vi "Get_Groups_And_Names.vi"(8 "error in (no error)":errorcluster, 11 "Constraints":T1 {"Estimate Quality" scale=0.0..5.0}) -> (0 "error out":errorcluster, 1 "Description":string[](array[string]), 2 "Groups":string[](array[string]), 3 "Names":string[](array[string]), 4 "Description Returned?":bool, 5 "Run start integer timestamp":i64[](array[numeric]), 6 "Run Time (hrs)":string[](array[string]), 7 "Run stop integer timestamp":i64[](array[numeric]))   [LabVIEW 2013]
uses:
  Constraints.ctl
  <vilib>/addons/database/Auxilliary.llb/DB Tools Cursor Type.ctl
  <vilib>/addons/database/Connection.llb/Conn Execute.vi
  <vilib>/addons/database/Recordset.llb/Rec Fetch Recordset Data (R).vi
  <userlib>/_OpenG.lib/array/array.llb/Empty 2D Array (Variant)__ogtk.vi
  <vilib>/addons/database/Recordset.llb/Rec Destroy - Connection.vi
  <userlib>/_OpenG.lib/array/array.llb/Remove Duplicates from 1D Array (String)__ogtk.vi
  <vilib>/addons/database/_DB Variant To Data/Database Variant To Data.xnode
  <vilib>/addons/database/NI_Database_API.lvlib
panel:
  out "SQL Lower Settings Query":string
  out "SQL Upper Settings Query":string
  out "Names SQL Query":string
  out "Groups SQL Query":string
  out "resulting string":string
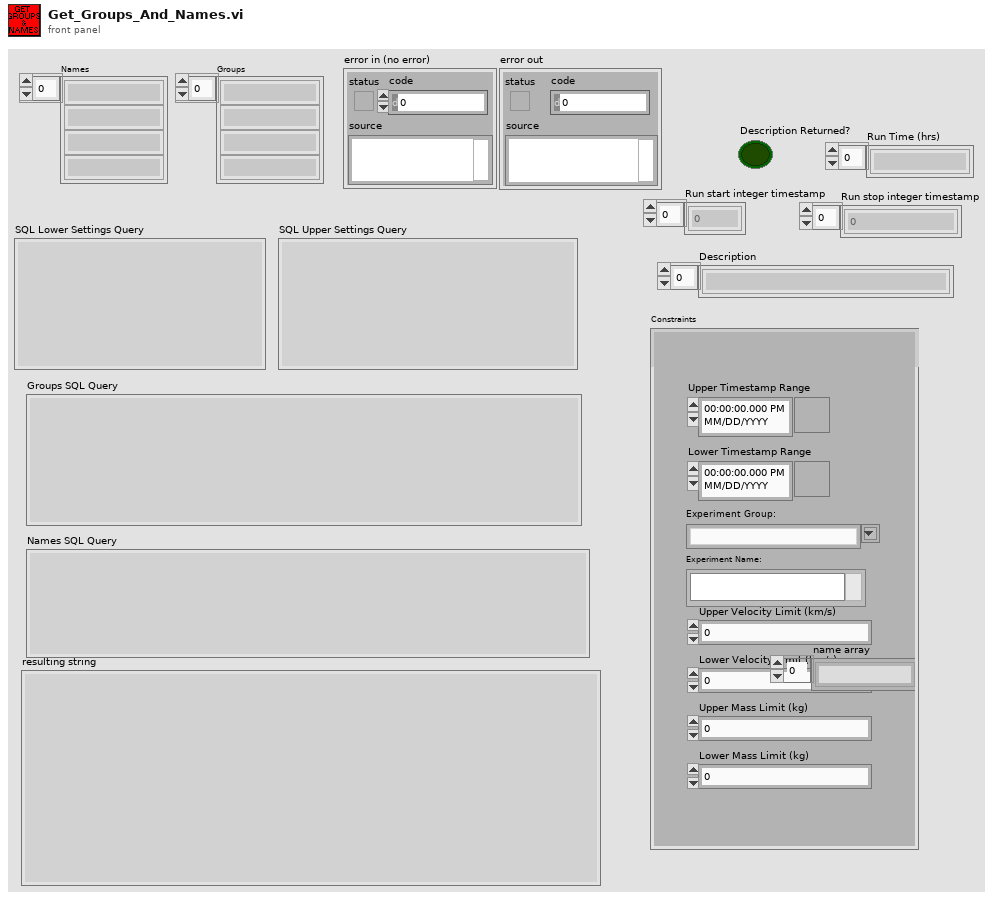
[diagram p1: front panel]
types:
  T1 = typedef "Constraints.ctl" = cluster{"Upper Timestamp Range":timestamp, "Lower Timestamp Range":timestamp, "Experiment Group:":string, "Experiment Name:":i32[], "Upper Velocity Limit (km/s)":dbl, "Lower Velocity Limit (km/s)":dbl, "Upper Mass Limit (kg)":dbl, "Lower Mass Limit (kg)":dbl, "name array":string[], "Estimate Quality":cluster{dbl, dbl}}
  T2 = typedef "NI_Database_API.lvlib/DB Tools Cursor Type.ctl" = enum16{"forward-only", "keyset", "dynamic", "static"}
  T3 = typedef "NI_Database_API.lvlib/Conn ObjectReference.ctl" = refnum<k1>
  T4 = typedef "NI_Database_API.lvlib/Rec ObjectReference.ctl" = refnum<k1>
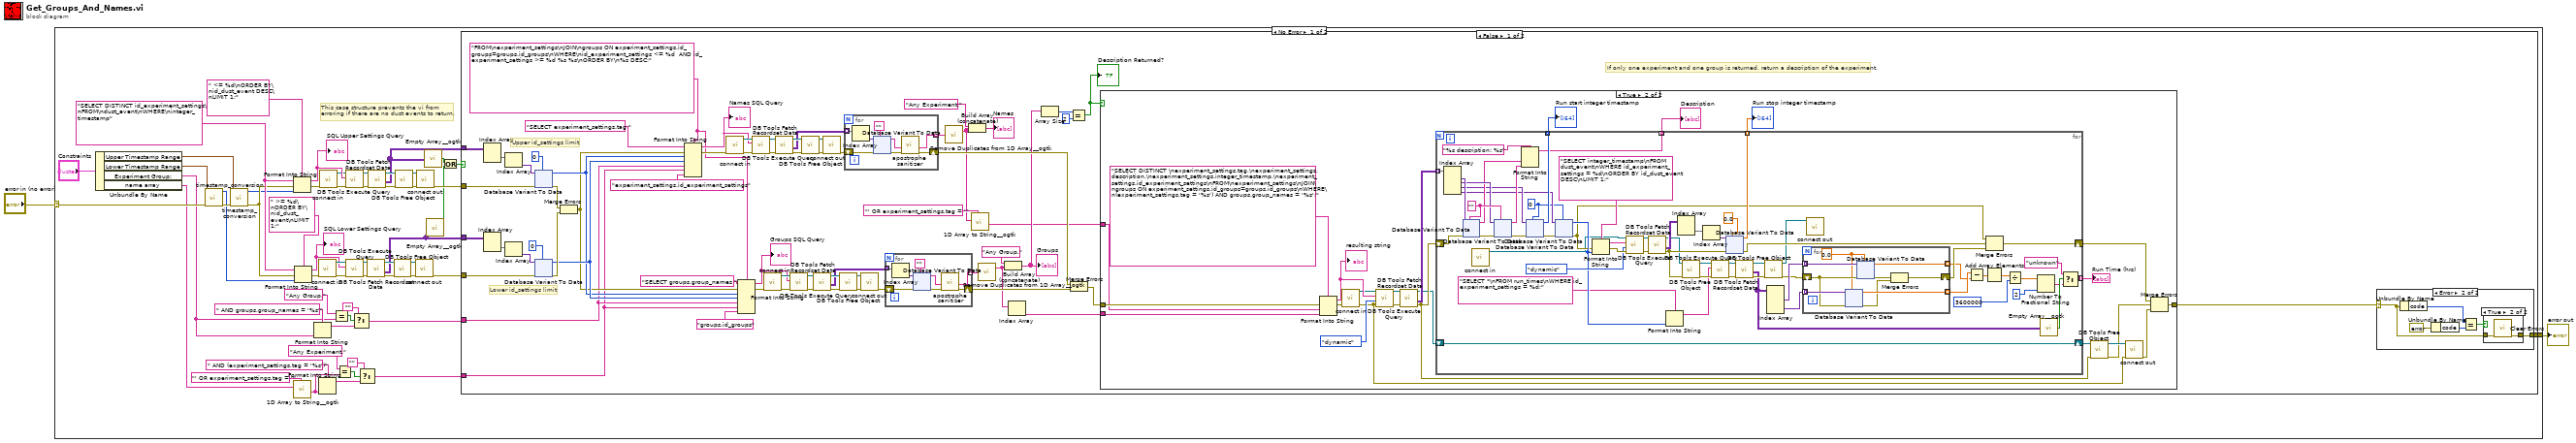
[diagram p0: block diagram]
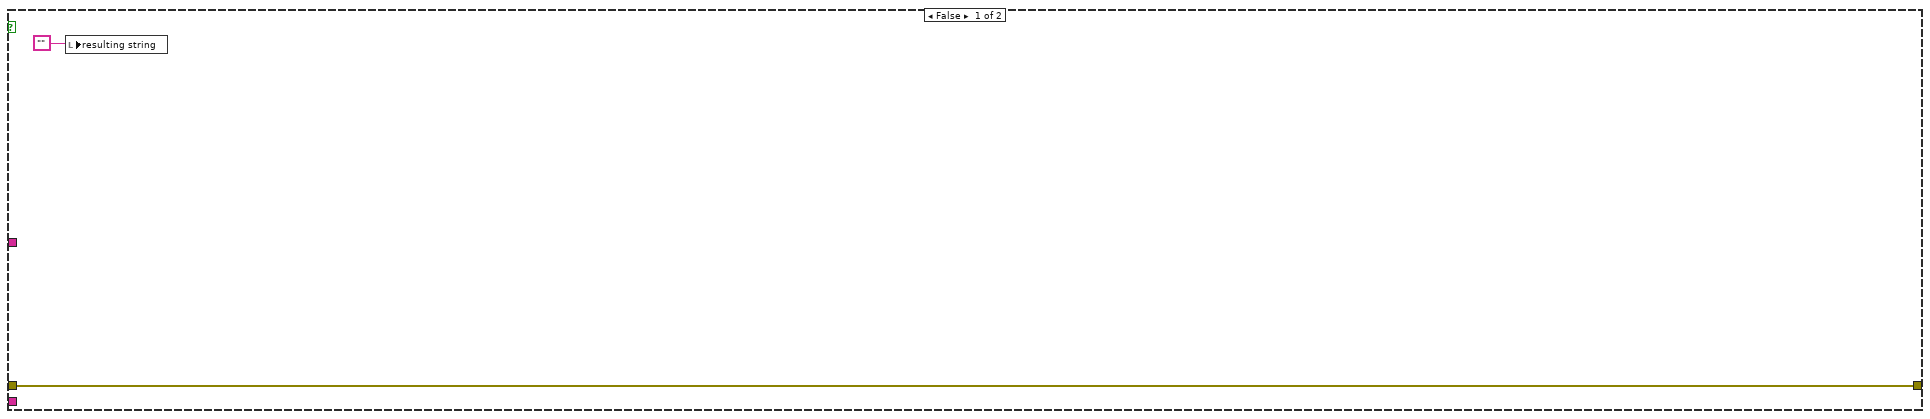
[diagram p4: hidden frame]
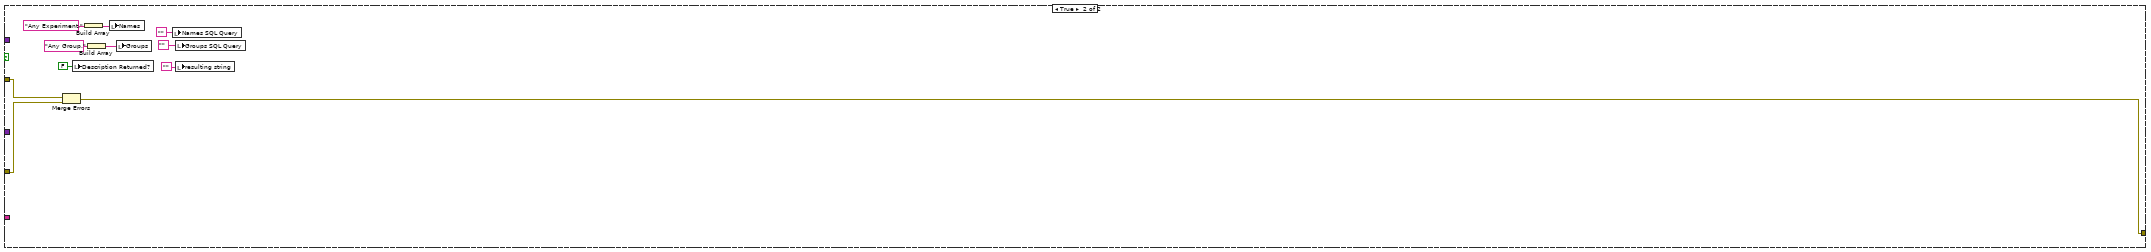
[diagram p5: hidden frame]
diagram:
  n1 = case shown="No Error" "error in (no error)" {
    selector: "error in (no error)" -> [w53 w607]
    tunnel: [w57 w607] -> w2
    frame No Error {
      w49 = "SELECT DISTINCT id_experiment_settings\nFROM\ndust_event\nWHERE\ninteger_timestamp" ("format string")
      # "This case structure prevents the vi from\nerroring if there are no dust events to return."
      n2 = Unbundle By Name("Constraints") -> ("Upper Timestamp Range"=w54:timestamp, "Lower Timestamp Range"=w55:timestamp, "Experiment Group:"=w6:string, "name array"=w23:string[])
      n3 = call "timestamp_conversion.vi"("error in (no error)"=w53, "Time Stamp"=w55) -> ("error out"=w56:errorcluster, "Integer Time"=w24:i64)  [unwired: 7 in]
      n4 = call "timestamp_conversion.vi"("error in (no error)"=w56, "Time Stamp"=w54) -> ("error out"=w26:errorcluster, "Integer Time"=w25:i64)  [unwired: 7 in]
      n5 = Format Into String(format string=" <= %d\nORDER BY\nid_dust_event DESC\nLIMIT 1;", initial string=w49, error in=w26, w25) -> (resulting string=w47:string, error out=w48:errorcluster)
      "SQL Upper Settings Query" <- w47
      n6 = call <userlib>:"1D Array to String__ogtk.vi"("delimiter (Tab)"="' OR experiment_settings.tag = '" ("string"), "Array of Strings"=w23) -> ("delimited string"=w5:string)  [unwired: 9 in]
      n7 = Format Into String(format string=" >= %d\nORDER BY\nid_dust_event\nLIMIT 1;", initial string=w49, error in=w26, w24) -> (resulting string=w29:string, error out=w30:errorcluster)
      "SQL Lower Settings Query" <- w29
      n8 = Format Into String(format string=" AND groups.group_names = '%s'" ("string"), w6) -> (resulting string=w10:string)  [unwired: 2 in, 1 out]
      n9 = call "connect in.vi"("error in (no error)"=w30) -> ("error out"=w32:errorcluster, "Database Connection"=w31:T3)  [unwired: 6 in, 1 out]
      n10 = Format Into String(format string=" AND (experiment_settings.tag = '%s')" ("string"), w5) -> (resulting string=w12:string)  [unwired: 2 in, 1 out]
      n11 = call "connect in.vi"("error in (no error)"=w48) -> ("error out"=w45:errorcluster, "Database Connection"=w46:T3)  [unwired: 6 in, 1 out]
      n12 = Equal?(x="Any Group.", y=w6) -> (x = y?=w11:bool)
      n13 = Equal?(x="Any Experiment.", y=w5) -> (x = y?=w16:bool)
      n14 = call-poly <vilib>:"DB Tools Execute Query.vi"("error in (no error)"=w45, "SQL query"=w47, "connection reference"=w46) -> ("error out"=w43:errorcluster, "recordset reference"=w44:T4)  [unwired: 5 in]
      n15 = call-poly <vilib>:"DB Tools Execute Query.vi"("error in (no error)"=w32, "SQL query"=w29, "connection reference"=w31) -> ("error out"=w34:errorcluster, "recordset reference"=w33:T4)  [unwired: 5 in]
      n16 = Select(t="", s=w11, f=w10) -> (s? t:f=w4:string)
      n17 = Select(t="", s=w16, f=w12) -> (s? t:f=w3:string)
      n18 = call-poly <vilib>:"DB Tools Fetch Recordset Data.vi"("error in (no error)"=w34, "recordset reference"=w33) -> ("error out"=w35:errorcluster, "recordset data"=w17:variant[][], "recordset reference out"=w36:T4)  [unwired: 3 in]
      n19 = call-poly <vilib>:"DB Tools Fetch Recordset Data.vi"("error in (no error)"=w43, "recordset reference"=w44) -> ("error out"=w42:errorcluster, "recordset data"=w18:variant[][], "recordset reference out"=w41:T4)  [unwired: 3 in]
      n20 = call-poly <vilib>:"DB Tools Free Object.vi"("error in (no error)"=w35, "recordset reference"=w36) -> ("error out"=w37:errorcluster, "connection reference"=w38:T3)  [unwired: 8 in]
      n21 = call-poly <vilib>:"DB Tools Free Object.vi"("error in (no error)"=w42, "recordset reference"=w41) -> ("error out"=w40:errorcluster, "connection reference"=w39:T3)  [unwired: 8 in]
      n22 = call "connect out.vi"("error in (no error)"=w37, "connection reference"=w38) -> ("error out"=w28:errorcluster)  [unwired: 9 in]
      n23 = call "connect out.vi"("error in (no error)"=w40, "connection reference"=w39) -> ("error out"=w27:errorcluster)  [unwired: 9 in]
      n24 = call-poly <userlib>:"Empty Array__ogtk.vi"("Array"=w18) -> ("Empty Array?"=w19:bool)  [unwired: 8 in]
      n25 = call-poly <userlib>:"Empty Array__ogtk.vi"("Array"=w17) -> ("Empty Array?"=w20:bool)  [unwired: 8 in]
      n26 = Or(x=w19, y=w20) -> (x .or. y?=w21:bool)
      n27 = case shown="False" w21 {
        tunnel: [w122 w604] -> w57
        tunnel: w18 -> [w119 _]
        tunnel: w17 -> [w118 _]
        tunnel: w28 -> [w117 w606]
        tunnel: w27 -> [w113 w605]
        tunnel: w4 -> [w66 _]
        tunnel: w3 -> [w65 _]
        frame False {
          w64 = "FROM\nexperiment_settings\nJOIN\ngroups ON experiment_settings.id_groups=groups.id_groups\nWHERE\nid_experiment_settings <= %d  AND id_experiment_settings >= %d %s %s\nORDER BY\n%s DESC;" ("string")
          # "Upper id_settings limit"
          # "Lower id_settings limit"
          # "If only one experiment and one group is returned, return a description of the experiment."
          n28 = Index Array(array=w118) -> (element=w120:variant[])  [unwired: 2 in]
          n29 = Index Array(array=w119) -> (element=w121:variant[])  [unwired: 2 in]
          n30 = Index Array(array=w120) -> (element=w116:variant)  [unwired: 1 in]
          n31 = Index Array(array=w121) -> (element=w112:variant)  [unwired: 1 in]
          n32 = xnode "Database Variant To Data"("database variant"=w112, "error in (no error)"=w113, "type"=0) -> ("data"=w108:i32, "error out"=w110:errorcluster)
          n33 = xnode "Database Variant To Data"("database variant"=w116, "error in (no error)"=w117, "type"=0) -> ("data"=w109:i32, "error out"=w111:errorcluster)
          n34 = Merge Errors(w110, w111) -> (w71:errorcluster)
          n35 = Format Into String(format string=w64, initial string="SELECT experiment_settings.tag ", error in=w71, w108, w109, w66, w65, "experiment_settings.id_experiment_settings") -> (resulting string=w79:string, error out=w88:errorcluster)
          "Names SQL Query" <- w79
          n36 = call "connect in.vi"("error in (no error)"=w88) -> ("error out"=w105:errorcluster, "Database Connection"=w106:T3)  [unwired: 6 in, 1 out]
          n37 = Format Into String(format string=w64, initial string="SELECT groups.group_names ", error in=w71, w108, w109, w66, w65, "groups.id_groups") -> (resulting string=w89:string, error out=w90:errorcluster)
          "Groups SQL Query" <- w89
          n38 = call-poly <vilib>:"DB Tools Execute Query.vi"("error in (no error)"=w105, "SQL query"=w79, "connection reference"=w106) -> ("error out"=w103:errorcluster, "recordset reference"=w104:T4)  [unwired: 5 in]
          n39 = call "connect in.vi"("error in (no error)"=w90) -> ("error out"=w92:errorcluster, "Database Connection"=w91:T3)  [unwired: 6 in, 1 out]
          n40 = call-poly <vilib>:"DB Tools Fetch Recordset Data.vi"("error in (no error)"=w103, "recordset reference"=w104) -> ("error out"=w102:errorcluster, "recordset data"=w87:variant[][], "recordset reference out"=w101:T4)  [unwired: 3 in]
          n41 = call-poly <vilib>:"DB Tools Execute Query.vi"("error in (no error)"=w92, "SQL query"=w89, "connection reference"=w91) -> ("error out"=w94:errorcluster, "recordset reference"=w93:T4)  [unwired: 5 in]
          n42 = call-poly <vilib>:"DB Tools Free Object.vi"("error in (no error)"=w102, "recordset reference"=w101) -> ("error out"=w100:errorcluster, "connection reference"=w99:T3)  [unwired: 8 in]
          n43 = call-poly <vilib>:"DB Tools Fetch Recordset Data.vi"("error in (no error)"=w94, "recordset reference"=w93) -> ("error out"=w95:errorcluster, "recordset data"=w81:variant[][], "recordset reference out"=w96:T4)  [unwired: 3 in]
          n44 = call "connect out.vi"("error in (no error)"=w100, "connection reference"=w99) -> ("error out"=w107:errorcluster)  [unwired: 9 in]
          n45 = call-poly <vilib>:"DB Tools Free Object.vi"("error in (no error)"=w95, "recordset reference"=w96) -> ("error out"=w97:errorcluster, "connection reference"=w98:T3)  [unwired: 8 in]
          n46 = for {
            tunnel: w87 -> [w167] mode=indexing
            tunnel: [w164] -> w85 mode=indexing
            shift-right: [w163] -> w80
            shift-left: w107 -> [w170]
            n47 = Index Array(array=w167) -> (element=w168:variant)  [unwired: 1 in]
            n48 = xnode "Database Variant To Data"("database variant"=w168, "error in (no error)"=w170, "type"="" ("t")) -> ("data"=w165:string, "error out"=w166:errorcluster)
            n49 = call "apostrophe sanitizer.vi"("error in (no error)"=w166, "result from db"=w165) -> ("error out"=w163:errorcluster, "fixed result from db"=w164:string)  [unwired: 7 in, 1 out]
          }
          n50 = call "connect out.vi"("error in (no error)"=w97, "connection reference"=w98) -> ("error out"=w82:errorcluster)  [unwired: 9 in]
          n51 = for {
            tunnel: w81 -> [w127] mode=indexing
            tunnel: [w124] -> w84 mode=indexing
            shift-right: [w123] -> w78
            shift-left: w82 -> [w130]
            n52 = Index Array(array=w127) -> (element=w128:variant)  [unwired: 1 in]
            n53 = xnode "Database Variant To Data"("database variant"=w128, "error in (no error)"=w130, "type"="" ("t")) -> ("data"=w125:string, "error out"=w126:errorcluster)
            n54 = call "apostrophe sanitizer.vi"("error in (no error)"=w126, "result from db"=w125) -> ("error out"=w123:errorcluster, "fixed result from db"=w124:string)  [unwired: 7 in, 1 out]
          }
          n55 = call-poly <userlib>:"Remove Duplicates from 1D Array__ogtk.vi"("Input Array"=w85) -> ("Output Array"=w59:string[])  [unwired: 1 out]
          n56 = Build Array (concatenate)("Any Experiment.", w59) -> (→"Names":string[])
          n57 = call <userlib>:"1D Array to String__ogtk.vi"("delimiter (Tab)"="' OR experiment_settings.tag = '" ("string"), "Array of Strings"=w59) -> ("delimited string"=w58:string)  [unwired: 9 in]
          n58 = call-poly <userlib>:"Remove Duplicates from 1D Array__ogtk.vi"("Input Array"=w84) -> ("Output Array"=w63:string[])  [unwired: 1 out]
          n59 = Build Array (concatenate)("Any Group.", w63) -> (w74:string[])
          "Groups" <- w74
          n60 = Index Array(array=w63) -> (element=w62:string)  [unwired: 1 in]
          n61 = Array Size(array=w74) -> (size(s)=w75:i32)
          n62 = Equal?(x=w75, y=2) -> (x = y?=w61:bool)
          "Description Returned?" <- w61
          n63 = Merge Errors(w80, w78) -> (w77:errorcluster)
          n64 = case shown="True" w61 {
            tunnel: w77 -> [w278 w290]
            tunnel: [w278 w292] -> w76
            tunnel: w62 -> [_ w280]
            tunnel: w58 -> [_ w279]
            frame False {
              n65 = local write "resulting string"("") -> ()
            }
            frame True {
              n66 = Format Into String(format string="SELECT DISTINCT \nexperiment_settings.tag,\nexperiment_settings.description,\nexperiment_settings.integer_timestamp,\nexperiment_settings.id_experiment_settings\nFROM\nexperiment_settings\nJOIN\ngroups ON experiment_settings.id_groups=groups.id_groups\nWHERE\n(experiment_settings.tag = '%s') AND groups.group_names = '%s';" ("string"), error in=w290, w279, w280) -> (resulting string=w298:string, error out=w297:errorcluster)  [unwired: 1 in]
              "resulting string" <- w298
              n67 = call "connect in.vi"("error in (no error)"=w297) -> ("error out"=w291:errorcluster, "Database Connection"=w285:T3)  [unwired: 6 in, 1 out]
              n68 = call-poly <vilib>:"DB Tools Execute Query.vi"("error in (no error)"=w291, "cursor type"=DB_Tools_Cursor_Type."dynamic", "SQL query"=w298, "connection reference"=w285) -> ("error out"=w302:errorcluster, "recordset reference"=w301:T4)  [unwired: 4 in]
              n69 = call-poly <vilib>:"DB Tools Fetch Recordset Data.vi"("error in (no error)"=w302, "recordset reference"=w301) -> ("error out"=w293:errorcluster, "recordset data"=w296:variant[][], "recordset reference out"=w289:T4)  [unwired: 3 in]
              n70 = for {
                shift-right: [w330] -> w287
                shift-left: w293 -> [w343]
                tunnel: w296 -> [w361] mode=indexing
                tunnel: [w353] -> w294 mode=indexing
                tunnel: [w351] -> w295 mode=indexing
                tunnel: [w335] -> w284 mode=indexing
                shift-right: [w334] -> w288
                shift-left: w289 -> [w334]
                tunnel: [w311] -> w286 mode=indexing
                w341 = i64 0 ("Integer Time")
                w360 = ""
                n71 = Index Array(array=w361) -> (element #1=w362:variant, element #2=w359:variant, element #3=w352:variant, element #4=w350:variant)  [unwired: 4 in]
                n72 = xnode "Database Variant To Data"("database variant"=w362, "error in (no error)"=w343, "type"=w360) -> ("data"=w356:string, "error out"=w358:errorcluster)
                n73 = call "connect in.vi"() -> ("Database Connection"=w303:T3)  [unwired: 7 in, 2 out]
                n74 = xnode "Database Variant To Data"("database variant"=w359, "error in (no error)"=w358, "type"=w360) -> ("data"=w355:string, "error out"=w354:errorcluster)
                n75 = Format Into String(format string="%s description: %s", w356, w355) -> (resulting string=w351:string)  [unwired: 2 in, 1 out]
                n76 = xnode "Database Variant To Data"("database variant"=w352, "error in (no error)"=w354, "type"=w341) -> ("data"=w353:i64, "error out"=w336:errorcluster)
                n77 = xnode "Database Variant To Data"("database variant"=w350, "error in (no error)"=w336, "type"=w341) -> ("data"=w329:i64, "error out"=w306:errorcluster)
                n78 = Format Into String(format string="SELECT integer_timestamp\nFROM dust_event\nWHERE id_experiment_settings = %d\nORDER BY id_dust_event DESC\nLIMIT 1;", error in=w306, w329) -> (resulting string=w347:string, error out=w348:errorcluster)  [unwired: 1 in]
                n79 = call-poly <vilib>:"DB Tools Execute Query.vi"("error in (no error)"=w348, "cursor type"=DB_Tools_Cursor_Type."dynamic", "SQL query"=w347, "connection reference"=w303) -> ("error out"=w344:errorcluster, "recordset reference"=w345:T4)  [unwired: 4 in]
                n80 = call-poly <vilib>:"DB Tools Fetch Recordset Data.vi"("error in (no error)"=w344, "recordset reference"=w345) -> ("error out"=w338:errorcluster, "recordset data"=w342:variant[][], "recordset reference out"=w337:T4)  [unwired: 3 in]
                n81 = Format Into String(format string="SELECT *\nFROM run_times\nWHERE id_experiment_settings = %d;", w329) -> (resulting string=w323:string)  [unwired: 2 in, 1 out]
                n82 = Index Array(array=w342) -> (element=w340:variant[])  [unwired: 2 in]
                n83 = call-poly <vilib>:"DB Tools Free Object.vi"("error in (no error)"=w338, "recordset reference"=w337) -> ("error out"=w332:errorcluster, "connection reference"=w333:T3)  [unwired: 8 in]
                n84 = Index Array(array=w340) -> (element=w339:variant)  [unwired: 1 in]
                n85 = call-poly <vilib>:"DB Tools Execute Query.vi"("error in (no error)"=w332, "SQL query"=w323, "connection reference"=w333) -> ("error out"=w327:errorcluster, "recordset reference"=w328:T4)  [unwired: 5 in]
                n86 = xnode "Database Variant To Data"("database variant"=w339, "error in (no error)"=w338, "type"=0.0) -> ("data"=w335:dbl, "error out"=w331:errorcluster)
                n87 = call-poly <vilib>:"DB Tools Fetch Recordset Data.vi"("error in (no error)"=w327, "recordset reference"=w328) -> ("error out"=w325:errorcluster, "recordset data"=w315:variant[][], "recordset reference out"=w326:T4)  [unwired: 3 in]
                n88 = call-poly <vilib>:"DB Tools Free Object.vi"("error in (no error)"=w325, "recordset reference"=w326) -> ("error out"=w316:errorcluster, "connection reference"=w304:T3)  [unwired: 8 in]
                n89 = Index Array(array=w315) -> (element #1=w322:variant[], element #2=w321:variant[])  [unwired: 4 in]
                n90 = for {
                  tunnel: w322 -> [w371] mode=indexing
                  tunnel: w321 -> [w370] mode=indexing
                  tunnel: [w367] -> w309 mode=indexing
                  tunnel: [w369] -> w308 mode=indexing
                  shift-right: [w364] -> w310
                  shift-left: w316 -> [w368]
                  w363 = 0.0
                  n91 = xnode "Database Variant To Data"("database variant"=w370, "error in (no error)"=w368, "type"=w363) -> ("data"=w367:dbl, "error out"=w365:errorcluster)
                  n92 = xnode "Database Variant To Data"("database variant"=w371, "error in (no error)"=w368, "type"=w363) -> ("data"=w369:dbl, "error out"=w366:errorcluster)
                  n93 = Merge Errors(w366, w365) -> (w364:errorcluster)
                }
                n94 = call "connect out.vi"("connection reference"=w304) -> ()  [unwired: 10 in, 1 out]
                n95 = Subtract(x=w309, y=w308) -> (x-y=w307:dbl[])
                n96 = Merge Errors(w306, w331, w310) -> (w330:errorcluster)
                n97 = Add Array Elements(numeric array=w307) -> (sum=w320:dbl)
                n98 = Divide(x=w320, y=i64 3600000) -> (x/y=w318:dbl)
                n99 = Number To Fractional String(number=w318, precision (6)=i16 2) -> (F-format string=w313:string)  [unwired: 2 in]
                n100 = call-poly <userlib>:"Empty Array__ogtk.vi"("Array"=w315) -> ("Empty Array?"=w314:bool)  [unwired: 8 in]
                n101 = Select(t="unknown" ("f"), s=w314, f=w313) -> (s? t:f=w311:string)
              }
              "Run start integer timestamp" <- w294
              "Description" <- w295
              "Run stop integer timestamp" <- w284
              "Run Time (hrs)" <- w286
              n102 = call-poly <vilib>:"DB Tools Free Object.vi"("error in (no error)"=w293, "recordset reference"=w288) -> ("error out"=w282:errorcluster, "connection reference"=w300:T3)  [unwired: 8 in]
              n103 = call "connect out.vi"("error in (no error)"=w291, "connection reference"=w300) -> ("error out"=w283:errorcluster)  [unwired: 9 in]
              n104 = Merge Errors(w287, w282, w283) -> (w292:errorcluster)
            }
          }
          n105 = case shown="Error" w76 {
            selector: w76 -> [w267 w268]
            tunnel: [w267 w269] -> w122
            frame No Error {
            }
            frame Error {
              n106 = Unbundle By Name(w268) -> ("code"=w270:i32)
              n107 = Unbundle By Name(errorcluster {"status"=TRUE, "code"=1, "source"="\"NI_Database_API.lvlib:Rec Delete.vi\"<ERR>Object 0x000000 is not valid."} ("error out")) -> ("code"=w271:i32)
              n108 = Equal?(x=w270, y=w271) -> (x = y?=w273:bool)
              n109 = case shown="True" w273 {
                tunnel: [w274 w275] -> w269
                tunnel: w268 -> [w274 w276]
                frame False {
                }
                frame True {
                  n110 = call <vilib>:"Clear Errors.vi"("error in (no error)"=w276) -> ("error out"=w275:errorcluster)  [unwired: 6 in]
                }
              }
            }
          }
        }
        frame True {
          n111 = Merge Errors(w605, w606) -> (w604:errorcluster)
          n112 = local write "Description Returned?"(FALSE ("Description Returned?")) -> ()
          n113 = Build Array("Any Experiment.") -> (w599:string[])
          n114 = Build Array("Any Group.") -> (w598:string[])
          n115 = local write "Names"(w599) -> ()
          n116 = local write "Groups"(w598) -> ()
          n117 = local write "Names SQL Query"("") -> ()
          n118 = local write "Groups SQL Query"("") -> ()
          n119 = local write "resulting string"("") -> ()
        }
      }
    }
    frame Error {
    }
  }
  "error out" <- w2
